vi "myFreqTime.vi"(6 "测量周期数 n":u32=2 min=1 max=10, 7 "同步频率上限 f_tick_ref":u32=1 min=1 max=50, 9 "freqs rows":i32[][](array[numeric]), 10 "f_tick_min":u32, 11 "f_mes_max":u32) -> (0 "n_tbase":u32, 1 "n_samp":u64, 2 "f_tick":dbl, 3 "f_mes":i32, 4 "mem_size":u32, 5 "row报告":string)   [LabVIEW 2024]
doc: "根据 f_tick_min, f_mes_max, 计算 freqs_group 的每行对应的 t_mes, t_tick, n_samp, n_base。"
uses:
  93082141-71ac-4920-8f54-44157a0ea3fd.vi
  <vilib>/gmath/NI_Gmath.lvlib
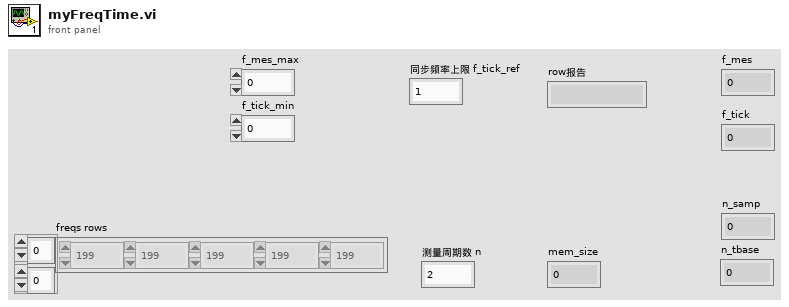
[diagram p1: front panel]
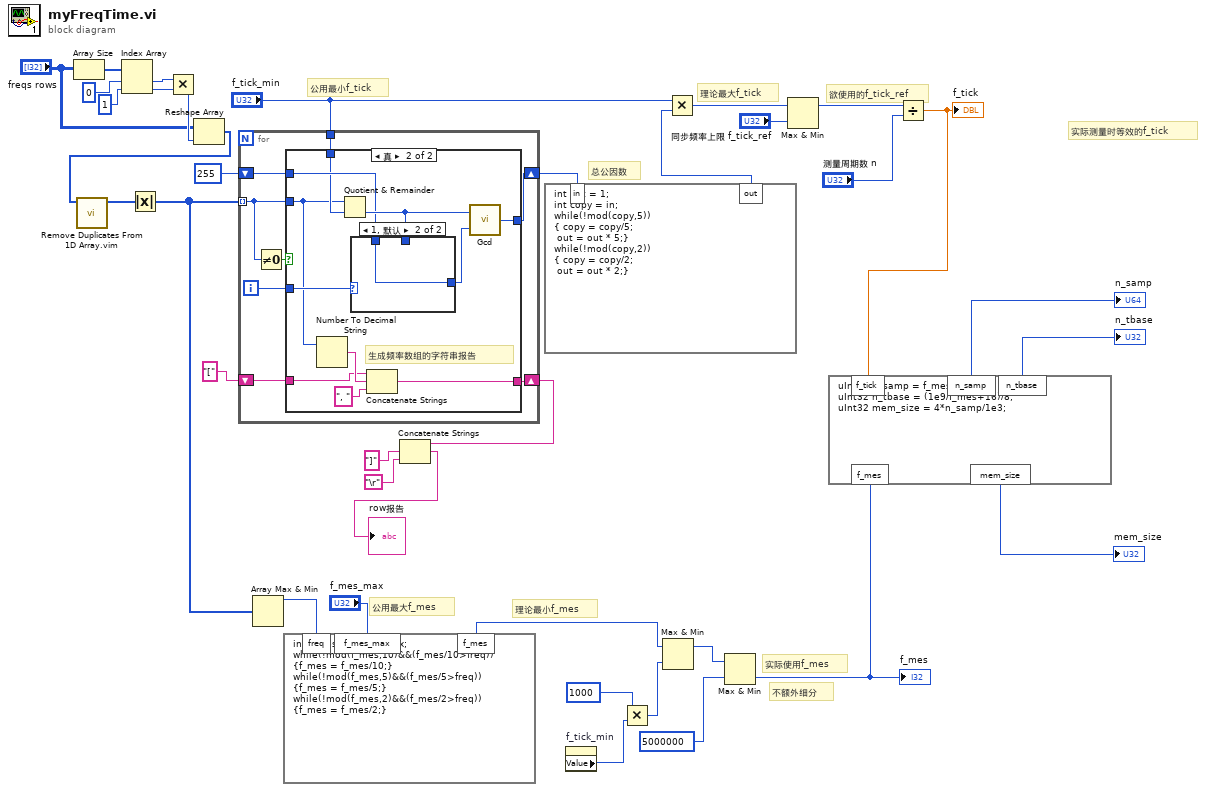
[diagram p0: block diagram]
diagram:
  # "不额外细分"
  # "公用最大f_mes"
  # "理论最小f_mes"
  # "实际测量时等效的f_tick"
  # "实际使用f_mes"
  # "公用最小f_tick"
  # "总公因数"
  # "欲使用的f_tick_ref"
  # "理论最大f_tick"
  n1 = Array Size(array="freqs rows") -> (size(s)=w8:i32[])
  n2 = Index Array(array=w8, index #1=0, index #2=1) -> (element #1=w5:i32, element #2=w4:i32)
  n3 = Multiply(x=w5, y=w4) -> (x*y=w3:i32)
  n4 = Reshape Array("freqs rows", w3) -> (w1:i32[])
  n5 = call "Remove Duplicates From 1D Array.vim"("array"=w1) -> ("array with duplicates removed"=w9:i32[])  [unwired: 10 in]
  n6 = Absolute Value(x=w9) -> (abs(x)=w10:i32[])
  n7 = for {
    tunnel: w10 -> [w38] mode=indexing
    shift-right: [w43] -> w25
    shift-left: 255 -> [w42]
    tunnel: "f_tick_min" -> [w39]
    shift-right: [w40] -> w29
    shift-left: "[" -> [w41]
    i -> [w44]
    n8 = Not Equal To 0?(x=w38) -> (x != 0?=w37:bool)
    n9 = case shown="真" w37 {
      tunnel: w44 -> [_ w57]
      tunnel: [w46 w54] -> w43
      tunnel: w42 -> [w46 w53]
      tunnel: w41 -> [w45 w50]
      tunnel: [w45 w49] -> w40
      tunnel: w39 -> [_ w48]
      tunnel: w38 -> [_ w47]
      frame False {
      }
      frame True {
        # "生成频率数组的字符串报告"
        n10 = Number To Decimal String(number=w47) -> (decimal integer string=w52:string)  [unwired: 1 in]
        n11 = Quotient & Remainder(x=w47, y=w48) -> (floor(x/y)=w56:u32)  [unwired: 1 out]
        n12 = case shown="1, 默认" w57 {
          tunnel: [w58 w59] -> w55
          tunnel: w56 -> [w58 _]
          tunnel: w53 -> [_ w59]
          frame 0 {
          }
          frame 1, Default {
          }
        }
        n13 = Concatenate Strings(w50, w52, ", ") -> (w49:string)
        n14 = call <vilib>:"Gcd.vi"("y"=w55, "x"=w56) -> ("gcd(x,y)"=w54:i32)
      }
    }
  }
  n15 = Array Max & Min(array=w10) -> (max value=w27:i32)  [unwired: 3 out]
  n16 = formula code="int f_mes = f_mes_max;\nwhile(!mod(f_mes,10)&&(f_mes/10>freq))\n{f_mes = f_mes/10;}\t\nwhile(!mod(f_mes,5)&&(f_mes/5>freq))\n{f_mes = f_mes/5;}\t\nwhile(!mod(f_mes,2)&&(f_mes/2>freq))\n{f_mes = f_mes/2;}"("freq"=w27, "f_mes_max"="f_mes_max") -> ("f_mes"=w19:i32)
  n17 = Concatenate Strings(w29, "]", "\r") -> (→"row报告":string)
  n18 = formula code="int out = 1;\nint copy = in;\nwhile(!mod(copy,5))\n{\tcopy = copy/5;\n\tout = out * 5;}\nwhile(!mod(copy,2))\n{\tcopy = copy/2;\n\tout = out * 2;}"("in"=w25) -> ("out"=w18:i32)
  n19 = property on="f_tick_min" class="DigNum (严格)"() -> ("Value"=w24:u32)  [unwired: 2 in, 2 out]
  n20 = Multiply(x=u32 1000, y=w24) -> (x*y=w22:u32)
  n21 = Max & Min(x=w19, y=w22) -> (max(x,y)=w21:u32)  [unwired: 1 out]
  n22 = Multiply(x="f_tick_min", y=w18) -> (x*y=w34:u32)
  n23 = Max & Min(x=w21, y=u32 5000000) -> (min(x,y)=w15:u32)  [unwired: 1 out]
  "f_mes" <- w15
  n24 = Max & Min(x=w34, y="同步频率上限 f_tick_ref") -> (max(x,y)=w17:u32)  [unwired: 1 out]
  n25 = Divide(x=w17, y="测量周期数 n") -> (x/y=w11:dbl)
  "f_tick" <- w11
  n26 = formula code="uInt32 n_samp = f_mes/f_tick;\nuInt32 n_tbase = (1e9/f_mes+16)/8;\nuInt32 mem_size = 4*n_samp/1e3;"("f_tick"=w11, "f_mes"=w15) -> ("n_samp"=→"n_samp":u32, "n_tbase"=→"n_tbase":u32, "mem_size"=→"mem_size":u32)
